vi "Asylum_Driver_GoToInitialPoint.vi"(6 "Abort Notifier":refnum<notifier>, 8 "error in (no error)":errorcluster, 9 "Z Setpoint":dbl, 10 "Coordinate":cluster{"X":dbl, "Y":dbl, "Speed":dbl}, 11 "Application":refnum<k7>) -> (0 "error out":errorcluster, 3 "Application":refnum<k7>)   [LabVIEW 2019]
uses:
  Asylum_Driver_XYMetersToVoltage.vi
  <userlib>/LevyLab/Igor API/private/Igor_NumericArraytoIgorWave.vi
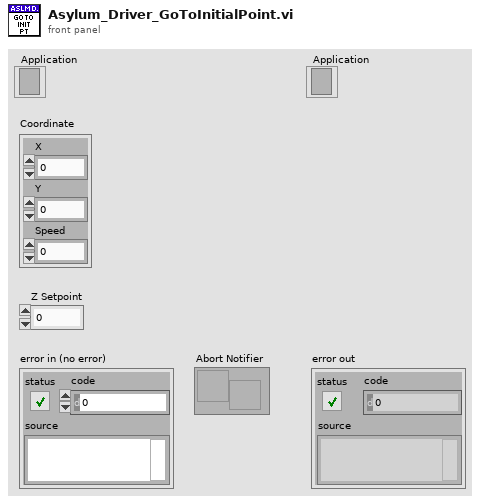
[diagram p1: front panel]
types:
  T1 = cluster{"setpoint":dbl, "pgain":dbl, "igain":dbl, "sgain":dbl}
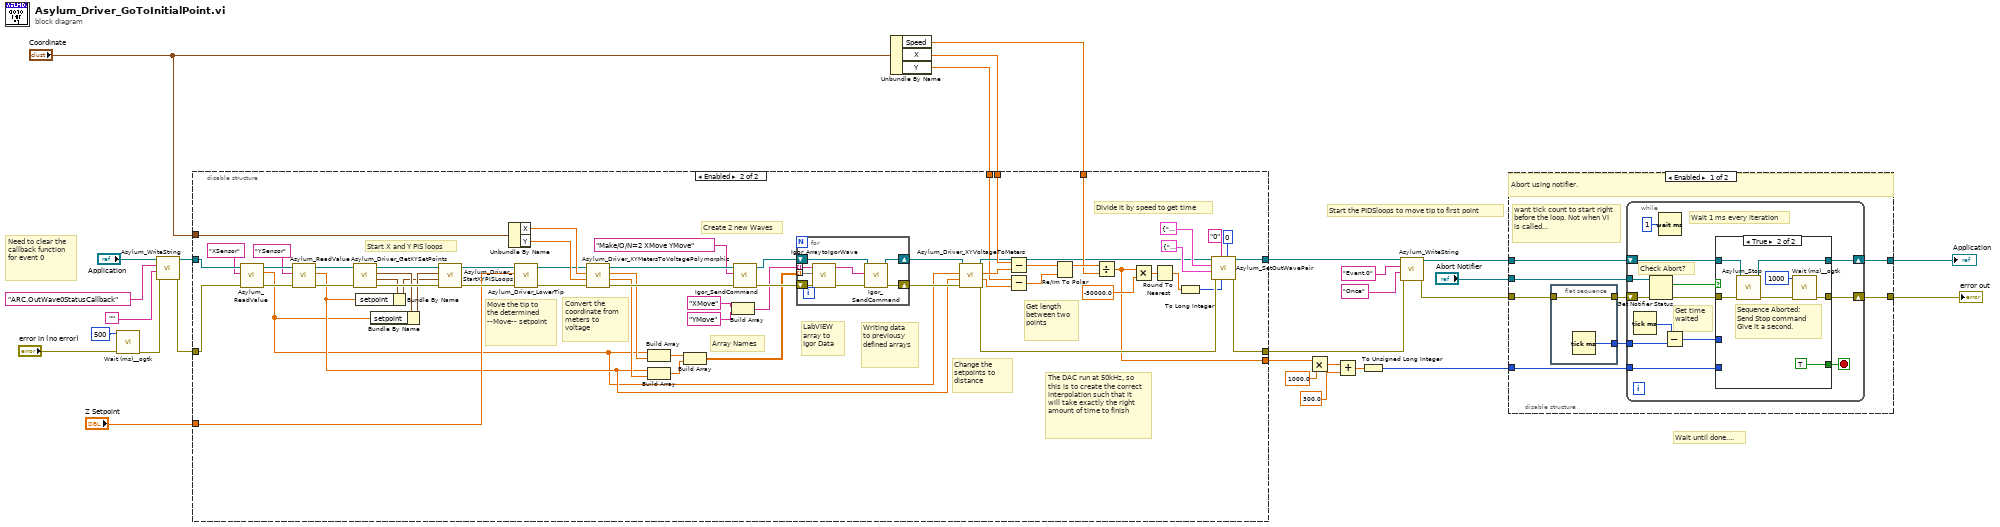
[diagram p0: block diagram]
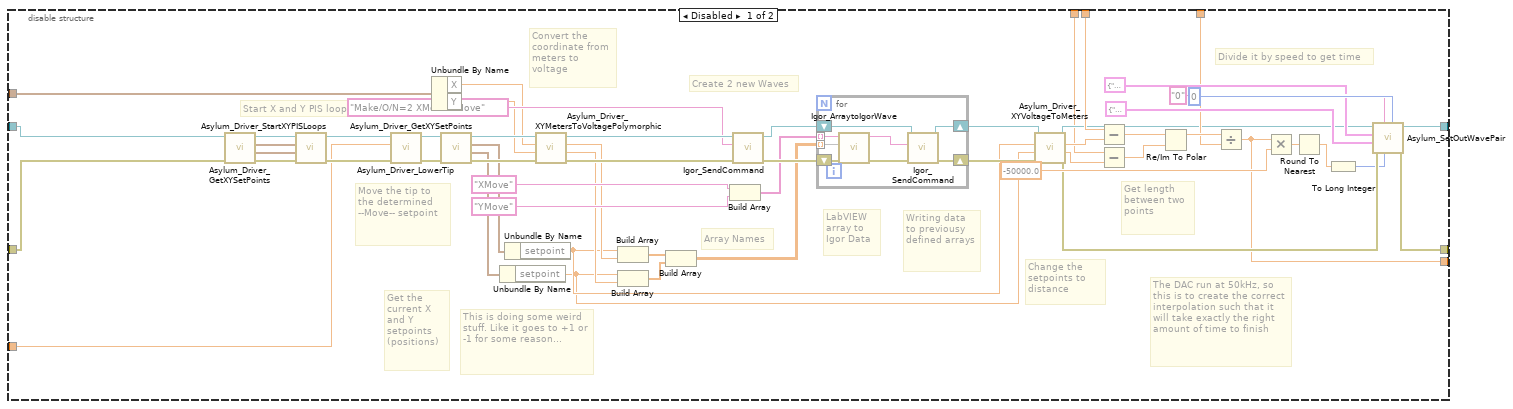
[diagram p2: hidden frame]
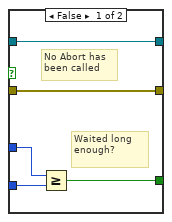
[diagram p3: hidden frame]
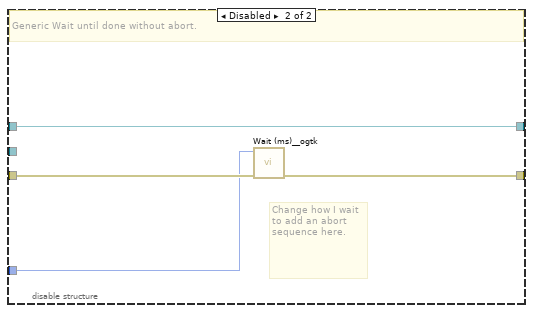
[diagram p4: hidden frame]
diagram:
  # "Wait until done...."
  # "Start the PIDSloops to move tip to first point"
  # "Need to clear the callback function for event 0"
  n1 = call <userlib>:"Wait (ms)__ogtk.vi"("error in (no error)"="error in (no error)", "milliseconds to wait"=u32 500) -> ("error out"=w24:errorcluster)  [unwired: 8 in, 1 out]
  n2 = call <userlib>:"Asylum_WriteString.vi"("error in (no error)"=w24, "valueString"="", "parameterName"="ARC.OutWave0StatusCallback", "Application"="Application") -> ("error out"=w1:errorcluster, "Application"=w4:refnum<k7>)  [unwired: 6 in]
  n3 = Unbundle By Name("Coordinate") -> ("Speed"=w15:dbl, "X"=w16:dbl, "Y"=w3:dbl)
  n4 = disable-structure shown="Enabled" {
    disable-tunnel: [w55 w127] -> w22
    disable-tunnel: [w54 w126] -> w20
    disable-tunnel: w16 -> [w52 w124]
    disable-tunnel: w15 -> [w50 w122]
    disable-tunnel: "Coordinate" -> [w48 w120]
    disable-tunnel: [w47 w119] -> w13
    disable-tunnel: w4 -> [w39 w106]
    disable-tunnel: w1 -> [w37 w105]
    disable-tunnel: w3 -> [w30 w110]
    disable-tunnel: "Z Setpoint" -> [w29 w109]
    frame Disabled {
      # "This is doing some weird stuff. Like it goes to +1 or -1 for some reason..."
      # "The DAC run at 50kHz, so this is to create the correct interpolation such that it will take exactly the right amount of time to finish"
      # "Divide it by speed to get time"
      # "Get length between two points"
      # "Change the setpoints to distance"
      # "Array Names"
      # "Writing data to previousy defined arrays"
      # "LabVIEW array to Igor Data"
      # "Create 2 new Waves"
      # "Convert the coordinate from meters to voltage"
      # "Get the current X and Y setpoints (positions)"
      # "Move the tip to the determined --Move-- setpoint"
      # "Start X and Y PIS loops"
      n5 = call "Asylum_Driver_GetXYSetPoints.vi"("error in (no error)"=w37, "Application"=w39) -> ("error out"=w36:errorcluster, "Y PIS Controls"=w34:T1, "X PIS Controls"=w35:T1, "Application"=w38:refnum<k7>)  [unwired: 6 in]
      n6 = call "Asylum_Driver_StartXYPISLoops.vi"("error in (no error)"=w36, "Y PIS Controls"=w34, "X PIS Controls"=w35, "Application"=w38) -> ("error out"=w80:errorcluster, "Application"=w84:refnum<k7>)  [unwired: 6 in]
      n7 = call "Asylum_Driver_LowerTip.vi"("error in (no error)"=w80, "Z Setpoint"=w29, "Application"=w84) -> ("error out"=w81:errorcluster, "Application"=w83:refnum<k7>)  [unwired: 7 in]
      n8 = Unbundle By Name(w48) -> ("X"=w49:dbl, "Y"=w51:dbl)
      n9 = call "Asylum_Driver_GetXYSetPoints.vi"("error in (no error)"=w81, "Application"=w83) -> ("error out"=w67:errorcluster, "Y PIS Controls"=w41:T1, "X PIS Controls"=w43:T1, "Application"=w82:refnum<k7>)  [unwired: 6 in]
      n10 = Unbundle By Name(w41) -> ("setpoint"=w40:dbl)
      n11 = Unbundle By Name(w43) -> ("setpoint"=w42:dbl)
      n12 = call-poly "Asylum_Driver_XYMetersToVoltagePolymorphic.vi"("error in (no error)"=w67, "Y Coordinate"=w51, "X Coordinate"=w49, "Application"=w82) -> ("error out"=w78:errorcluster, "Y Voltage"=w45:dbl, "X Voltage"=w46:dbl, "Application"=w79:refnum<k7>)  [unwired: 4 in]
      n13 = Build Array(w42, w46) -> (w76:dbl[])
      n14 = Build Array(w40, w45) -> (w75:dbl[])
      n15 = Build Array(w76, w75) -> (w70:dbl[][])
      n16 = Build Array("XMove", "YMove") -> (w71:string[])
      n17 = call <userlib>:"Igor_SendCommand.vi"("error in (no error)"=w78, "command"="Make/O/N=2 XMove YMove", "Application In"=w79) -> ("error out"=w72:errorcluster, "Application Out"=w69:refnum<k7>)  [unwired: 5 in, 2 out]
      n18 = for {
        tunnel: w71 -> [w90] mode=indexing
        tunnel: w70 -> [w89] mode=indexing
        shift-right: [w85] -> w31
        shift-left: w69 -> [w86]
        shift-right: [w88] -> w68
        shift-left: w72 -> [w92]
        n19 = call-poly <userlib>:"Igor_ArraytoIgorWave.vi"("error in (no error)"=w92, "Wave"=w89, "Name"=w90) -> ("error out"=w91:errorcluster, "Igor Wave"=w87:string)  [unwired: 7 in]
        n20 = call <userlib>:"Igor_SendCommand.vi"("error in (no error)"=w91, "command"=w87, "Application In"=w86) -> ("error out"=w88:errorcluster, "Application Out"=w85:refnum<k7>)  [unwired: 5 in, 2 out]
      }
      n21 = call "Asylum_Driver_XYVoltageToMeters.vi"("error in (no error)"=w68, "Y Voltage"=w40, "X Voltage"=w42, "Application"=w31) -> ("error out"=w60:errorcluster, "Y Meters"=w65:dbl, "X Meters"=w66:dbl, "Application"=w32:refnum<k7>)  [unwired: 4 in]
      n22 = Subtract(x=w52, y=w66) -> (x-y=w64:dbl)
      n23 = Subtract(x=w30, y=w65) -> (x-y=w63:dbl)
      n24 = Re/Im To Polar(2:w63, 3:w64) -> (1:w62:dbl)  [unwired: 1 out]
      n25 = Divide(x=w62, y=w50) -> (x/y=w47:dbl)
      n26 = Multiply(x=w47, y=-50000.0) -> (x*y=w53:dbl)
      n27 = Round To Nearest(number=w53) -> (nearest integer value=w33:dbl)
      n28 = To Long Integer(number=w33) -> (32bit integer=w44:i32)
      n29 = call <userlib>:"Asylum_SetOutWavePair.vi"("whichBank"=0, "interpolation"=w44, "eventString"="0", "error in (no error)"=w60, "Wave B"=cluster{"channelStringB":string, "waveB":string} {"channelStringB"="PIDSLoop.1.Setpoint", "waveB"="YMove"}, "Wave A"=cluster{"channelStringA":string, "waveA":string} {"channelStringA"="PIDSLoop.0.Setpoint", "waveA"="XMove"}, "Application"=w32) -> ("error out"=w54:errorcluster, "Application"=w55:refnum<k7>)  [unwired: 3 in]
    }
    frame Enabled {
      # "The DAC run at 50kHz, so this is to create the correct interpolation such that it will take exactly the right amount of time to finish"
      # "Divide it by speed to get time"
      # "Get length between two points"
      # "Change the setpoints to distance"
      # "Array Names"
      # "Writing data to previousy defined arrays"
      # "LabVIEW array to Igor Data"
      # "Create 2 new Waves"
      # "Convert the coordinate from meters to voltage"
      # "Move the tip to the determined --Move-- setpoint"
      # "Start X and Y PIS loops"
      n30 = call <userlib>:"Asylum_ReadValue.vi"("error in (no error)"=w105, "Value"="XSensor", "Application"=w106) -> ("error out"=w102:errorcluster, "Value"=w93:dbl, "Application"=w104:refnum<k7>)  [unwired: 6 in]
      n31 = call <userlib>:"Asylum_ReadValue.vi"("error in (no error)"=w102, "Value"="YSensor", "Application"=w104) -> ("error out"=w101:errorcluster, "Value"=w94:dbl, "Application"=w103:refnum<k7>)  [unwired: 6 in]
      n32 = call "Asylum_Driver_GetXYSetPoints.vi"("error in (no error)"=w101, "Application"=w103) -> ("error out"=w114:errorcluster, "Y PIS Controls"=w96:T1, "X PIS Controls"=w98:T1, "Application"=w115:refnum<k7>)  [unwired: 6 in]
      n33 = Bundle By Name(cluster=w96, "setpoint"=w94) -> (w95:T1)
      n34 = Bundle By Name(cluster=w98, "setpoint"=w93) -> (w97:T1)
      n35 = call "Asylum_Driver_StartXYPISLoops.vi"("error in (no error)"=w114, "Y PIS Controls"=w95, "X PIS Controls"=w97, "Application"=w115) -> ("error out"=w151:errorcluster, "Application"=w152:refnum<k7>)  [unwired: 6 in]
      n36 = Unbundle By Name(w120) -> ("X"=w121:dbl, "Y"=w123:dbl)
      n37 = call "Asylum_Driver_LowerTip.vi"("error in (no error)"=w151, "Z Setpoint"=w109, "Application"=w152) -> ("error out"=w107:errorcluster, "Application"=w108:refnum<k7>)  [unwired: 7 in]
      n38 = call-poly "Asylum_Driver_XYMetersToVoltagePolymorphic.vi"("error in (no error)"=w107, "Y Coordinate"=w123, "X Coordinate"=w121, "Application"=w108) -> ("error out"=w149:errorcluster, "Y Voltage"=w117:dbl, "X Voltage"=w118:dbl, "Application"=w150:refnum<k7>)  [unwired: 4 in]
      n39 = Build Array(w93, w118) -> (w147:dbl[])
      n40 = Build Array(w94, w117) -> (w146:dbl[])
      n41 = Build Array(w147, w146) -> (w141:dbl[][])
      n42 = Build Array("XMove", "YMove") -> (w142:string[])
      n43 = call <userlib>:"Igor_SendCommand.vi"("error in (no error)"=w149, "command"="Make/O/N=2 XMove YMove", "Application In"=w150) -> ("error out"=w143:errorcluster, "Application Out"=w140:refnum<k7>)  [unwired: 5 in, 2 out]
      n44 = for {
        tunnel: w142 -> [w158] mode=indexing
        tunnel: w141 -> [w157] mode=indexing
        shift-right: [w153] -> w111
        shift-left: w140 -> [w154]
        shift-right: [w156] -> w139
        shift-left: w143 -> [w160]
        n45 = call-poly <userlib>:"Igor_ArraytoIgorWave.vi"("error in (no error)"=w160, "Wave"=w157, "Name"=w158) -> ("error out"=w159:errorcluster, "Igor Wave"=w155:string)  [unwired: 7 in]
        n46 = call <userlib>:"Igor_SendCommand.vi"("error in (no error)"=w159, "command"=w155, "Application In"=w154) -> ("error out"=w156:errorcluster, "Application Out"=w153:refnum<k7>)  [unwired: 5 in, 2 out]
      }
      n47 = call "Asylum_Driver_XYVoltageToMeters.vi"("error in (no error)"=w139, "Y Voltage"=w94, "X Voltage"=w93, "Application"=w111) -> ("error out"=w132:errorcluster, "Y Meters"=w137:dbl, "X Meters"=w138:dbl, "Application"=w112:refnum<k7>)  [unwired: 4 in]
      n48 = Subtract(x=w124, y=w138) -> (x-y=w136:dbl)
      n49 = Subtract(x=w110, y=w137) -> (x-y=w135:dbl)
      n50 = Re/Im To Polar(2:w135, 3:w136) -> (1:w134:dbl)  [unwired: 1 out]
      n51 = Divide(x=w134, y=w122) -> (x/y=w119:dbl)
      n52 = Multiply(x=w119, y=-50000.0) -> (x*y=w125:dbl)
      n53 = Round To Nearest(number=w125) -> (nearest integer value=w113:dbl)
      n54 = To Long Integer(number=w113) -> (32bit integer=w116:i32)
      n55 = call <userlib>:"Asylum_SetOutWavePair.vi"("whichBank"=0, "interpolation"=w116, "eventString"="0", "error in (no error)"=w132, "Wave B"=cluster{"channelStringB":string, "waveB":string} {"channelStringB"="PIDSLoop.1.Setpoint", "waveB"="YMove"}, "Wave A"=cluster{"channelStringA":string, "waveA":string} {"channelStringA"="PIDSLoop.0.Setpoint", "waveA"="XMove"}, "Application"=w112) -> ("error out"=w126:errorcluster, "Application"=w127:refnum<k7>)  [unwired: 3 in]
    }
  }
  n56 = Multiply(x=w13, y=1000.0) -> (x*y=w18:dbl)
  n57 = Add(x=w18, y=300.0) -> (x+y=w11:dbl)
  n58 = To Unsigned Long Integer(number=w11) -> (unsigned 32bit integer=w10:u32)
  n59 = call <userlib>:"Asylum_WriteString.vi"("error in (no error)"=w20, "valueString"="Once", "parameterName"="Event.0", "Application"=w22) -> ("error out"=w9:errorcluster, "Application"=w6:refnum<k7>)  [unwired: 6 in]
  n60 = disable-structure shown="Enabled" {
    disable-tunnel: w9 -> [w167 w199]
    disable-tunnel: w10 -> [w162 w196]
    disable-tunnel: w6 -> [w164 w197]
    disable-tunnel: [w163 w197] -> w7
    disable-tunnel: [w166 w198] -> w8
    disable-tunnel: "Abort Notifier" -> [w161 _]
    frame Enabled {
      # "want tick count to start right before the loop. Not when VI is called..."
      # "Abort using notifier."
      n61 = flat-sequence {
        tunnel: [w169] -> w165
        tunnel: w167 -> [w170]
        tunnel: [w170] -> w168
        frame #0 {
          n62 = Tick Count (ms)() -> (millisecond timer value=w169:u32)
        }
      }
      n63 = while {
        tunnel: w161 -> [w180]
        shift-right: [w177] -> w163
        shift-left: w164 -> [w178]
        shift-right: [w182] -> w166
        shift-left: w168 -> [w181]
        tunnel: w165 -> [w174]
        tunnel: w162 -> [w171]
        stop <- w176 stop-if-true
        # "Check Abort?"
        # "Wait 1 ms every iteration"
        # "Get time waited"
        n64 = Tick Count (ms)() -> (millisecond timer value=w175:u32)
        n65 = Get Notifier Status(notifier=w180, error in (no error)=w181) -> (current notification=w179:bool, error out=w183:errorcluster)  [unwired: 3 out]
        n66 = Wait (ms)(milliseconds to wait=u32 1) -> ()  [unwired: 1 out]
        n67 = Subtract(x=w175, y=w174) -> (x-y=w172:u32)
        n68 = case shown="True" w179 {
          tunnel: w178 -> [w187 w194]
          tunnel: [w187 w193] -> w177
          tunnel: w183 -> [w188 w195]
          tunnel: [w188 w190] -> w182
          tunnel: [w184 TRUE] -> w176
          tunnel: w172 -> [w186 _]
          tunnel: w171 -> [w185 _]
          frame False {
            # "No Abort has been called"
            # "Waited long enough?"
            n69 = Greater Or Equal?(x=w186, y=w185) -> (x >= y?=w184:bool)
          }
          frame True {
            # "Sequence Aborted:\nSend Stop command\nGive it a second."
            n70 = call <userlib>:"Asylum_Stop.vi"("error in (no error)"=w195, "Application"=w194) -> ("error out"=w191:errorcluster, "Application"=w193:refnum<k7>)  [unwired: 8 in]
            n71 = call <userlib>:"Wait (ms)__ogtk.vi"("error in (no error)"=w191, "milliseconds to wait"=u32 1000) -> ("error out"=w190:errorcluster)  [unwired: 8 in, 1 out]
          }
        }
      }
    }
    frame Disabled {
      # "Change how I wait to add an abort sequence here."
      # "Generic Wait until done without abort."
      n72 = call <userlib>:"Wait (ms)__ogtk.vi"("error in (no error)"=w199, "milliseconds to wait"=w196) -> ("error out"=w198:errorcluster)  [unwired: 8 in, 1 out]
    }
  }
  "error out" <- w8
  "Application" <- w7
